vi "DI Coil UI.vi"(8 "error in (no error)":errorcluster, 11 "Node Ptr":T2 format="%.0x") -> (0 "error out":errorcluster)   [LabVIEW 2020, in "Modbus Master System Explorer.lvlib"]
uses:
  Modbus Master System Explorer.lvlib
  <vilib>/NI VeriStand/Custom Device API/Custom Device Item Ref.ctl
  SubVIs/Radix.ctl
  <vilib>/NI VeriStand/Custom Device API/Custom Device API.lvlib
panel:
  in  "Radix":T1
  in  "Valid?":string
  in  "Address":u16
  in  "Header":cluster{"Section Name":string}={"Section Name"="Discrete Input Settings"}
  in  "Description":string
  in  "Name":string
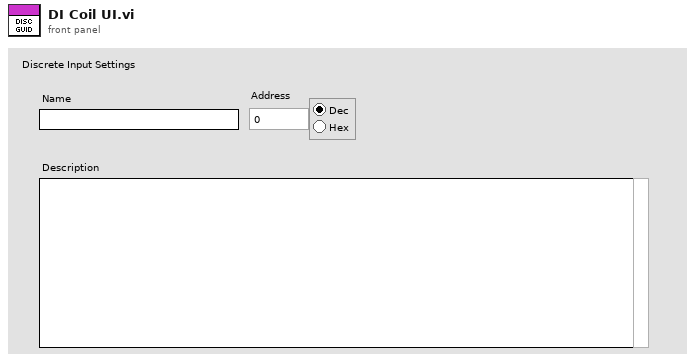
[diagram p1: front panel]
types:
  T1 = typedef "Modbus Master System Explorer.lvlib/Radix.ctl" = enum32{"Decimal", "Hexidecimal"}
  T2 = typedef "Custom Device API.lvlib/Custom Device Item Ref.ctl" = u64
  T3 = typedef "Custom Device API.lvlib/Custom Device Commands.ctl" = enum16{"Default", "Item renamed", "Shutdown", "Dynamic button pressed"}
  T4 = typedef "Custom Device API.lvlib/Custom Device Item Info.ctl" = cluster{"Name":string, "Is Channel":bool, "GUID":string, "Is Waveform":bool}
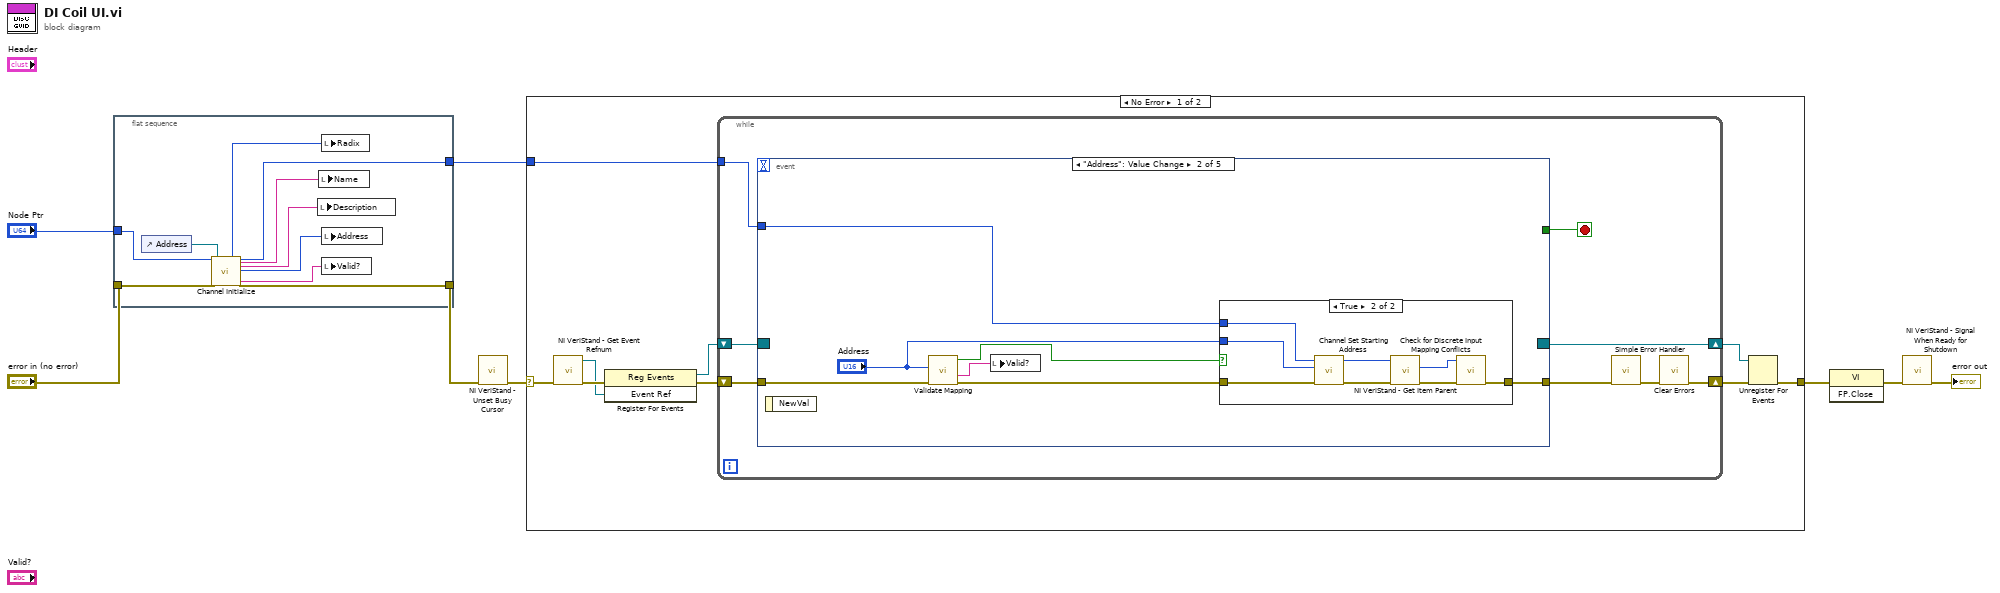
[diagram p0: block diagram]
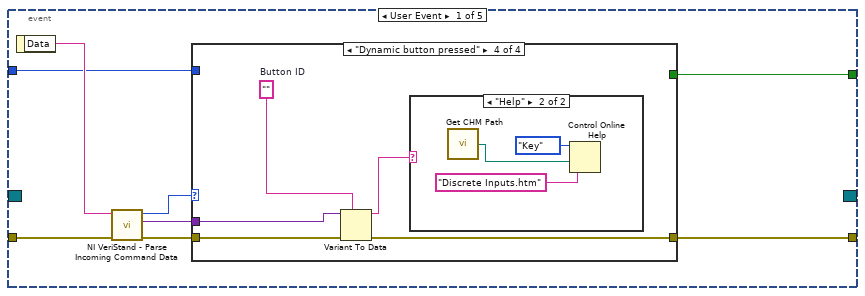
[diagram p2: hidden frame]
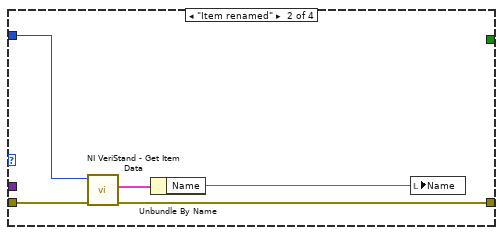
[diagram p4: hidden frame]
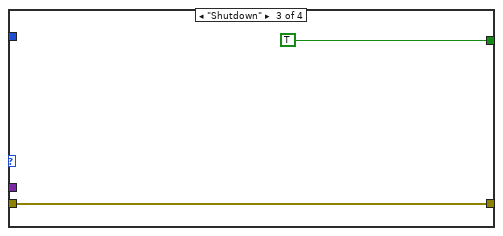
[diagram p5: hidden frame]
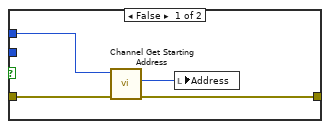
[diagram p7: hidden frame]
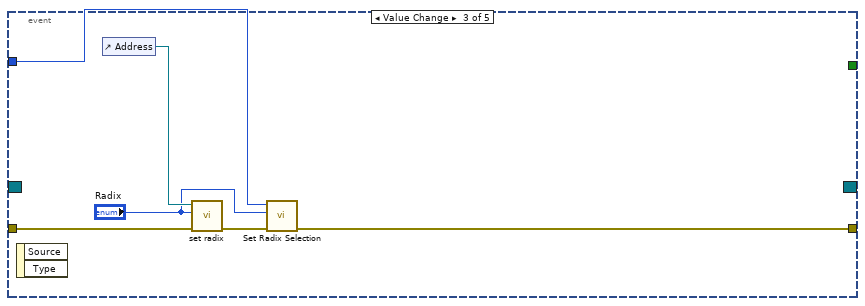
[diagram p8: hidden frame]
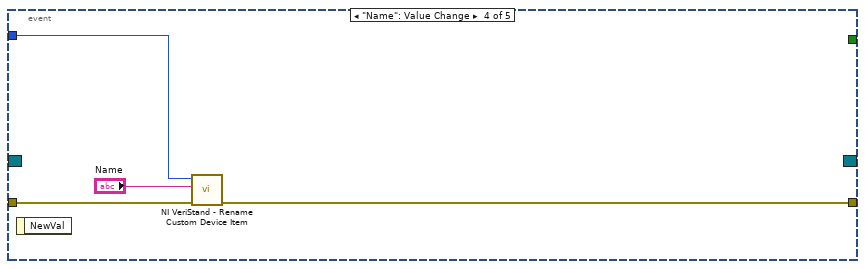
[diagram p9: hidden frame]
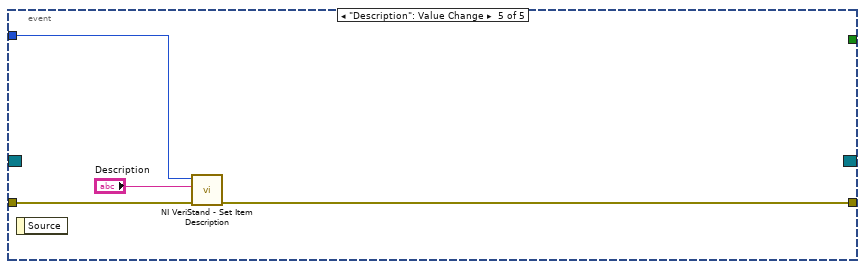
[diagram p10: hidden frame]
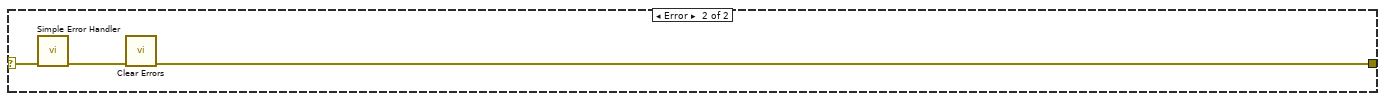
[diagram p11: hidden frame]
diagram:
  n1 = flat-sequence {
    tunnel: "Node Ptr" -> [w12]
    tunnel: [w11] -> w3
    tunnel: "error in (no error)" -> [w10]
    tunnel: [w9] -> w1
    frame #0 {
      n2 = control-ref of="Address"() -> (w17:refnum<vi>)
      n3 = call "Channel Initialize.vi"("Item Ref in"=w12, "error in (no error)"=w10, "Starting Address Ref in"=w17) -> ("Radix"=w18:T1, "Channel Ref out"=w11:T2, "Name"=w15:string, "Description"=w13:string, "Starting Address"=w14:u16, "Status Message"=w16:string, "error out"=w9:errorcluster)  [unwired: 12 in, 6 out]
      n4 = local write "Description"(w13) -> ()
      n5 = local write "Name"(w15) -> ()
      n6 = local write "Radix"(w18) -> ()
      n7 = local write "Address"(w14) -> ()
      n8 = local write "Valid?"(w16) -> ()
    }
  }
  n9 = call <vilib>:"NI VeriStand - Unset Busy Cursor.vi"("error in (no error)"=w1) -> ("error out"=w5:errorcluster)  [unwired: 10 out]
  n10 = case shown="No Error" w5 {
    selector: w5 -> [w19 w95]
    tunnel: [w24 w93] -> w8
    tunnel: w3 -> [w20 _]
    frame No Error {
      n11 = call <vilib>:"NI VeriStand - Get Event Refnum.vi"("error in (no error)"=w19) -> ("error out"=w27:errorcluster, "Event Ref"=w23:refnum<user-event>)  [unwired: 9 out]
      n12 = register-events(error in=w27, w23) -> (reference out=w21:refnum<event-registration>, error out=w22:errorcluster)  [unwired: 1 in]
      n13 = while {
        tunnel: w20 -> [w31]
        shift-right: [w28] -> w25
        shift-left: w22 -> [w34]
        shift-right: [w35] -> w26
        shift-left: w21 -> [w33]
        stop <- w32 stop-if-true
        n14 = event shown="[1] \"Address\": Value Change" {
          selector: w33 -> [_ _ _ _ _]
          dyn-events: [_ _ _ _ _] -> w35
          timeout: _ -> [_ _ _ _ _]
          tunnel: w34 -> [w43 w62 w83 w88 w91]
          tunnel: [w39 _ _ _ _] -> w32
          tunnel: [w38 w64 w80 w87 w90] -> w30
          tunnel: w31 -> [w37 w66 w81 w86 w92]
          event User Event {
            n15 = event-data() -> ("Data"=w42:string)  [unwired: 1 out]
            n16 = call <vilib>:"NI VeriStand - Parse Incoming Command Data.vi"("error in (no error)"=w43, "Incoming data"=w42) -> ("error out"=w41:errorcluster, "Outgoing data"=w36:variant, "Action"=w40:T3)  [unwired: 7 out]
            n17 = case shown="\"Dynamic button pressed\"" w40 {
              tunnel: w41 -> [w44 w49 w50 w56]
              tunnel: [_ _ TRUE _] -> w39
              tunnel: [w44 w46 w50 w53] -> w38
              tunnel: w37 -> [_ w48 _ _]
              tunnel: w36 -> [_ _ _ w55]
              frame "Default", Default {
              }
              frame "Item renamed" {
                n18 = call <vilib>:"NI VeriStand - Get Item Data.vi"("error in (no error)"=w49, "Item Ref in"=w48) -> ("error out"=w46:errorcluster, "Item Info"=w47:T4)  [unwired: 8 out]
                n19 = Unbundle By Name(w47) -> ("Name"=w45:string)
                n20 = local write "Name"(w45) -> ()
              }
              frame "Shutdown" {
              }
              frame "Dynamic button pressed" {
                w54 = ""  # Button ID
                n21 = Variant To Data(error in=w56, type=w54, Variant=w55) -> (data=w52:string, error out=w53:errorcluster)
                n22 = case shown="\"Help\"" w52 {
                  frame Default {
                  }
                  frame "Help" {
                    n23 = call "Get CHM Path.vi"() -> ("appended path"=w59:path)
                    n24 = Control Online Help(2:w59, 3:"Discrete Inputs.htm" ("String to search for"), 4:enum16{"Contents", "Key", "Close"}."Key" ("Operation")) -> ()  [unwired: 1 in, 1 out]
                  }
                }
              }
            }
          }
          event "Address": Value Change {
            n25 = event-data() -> ()  [unwired: 2 out]
            n26 = call "Validate Mapping.vi"("error in (no error)"=w62, "Mapping"="Address") -> ("error out"=w61:errorcluster, "Status Message"=w60:string, "Valid?"=w63:bool)  [unwired: 7 in]
            n27 = local write "Valid?"(w60) -> ()
            n28 = case shown="True" w63 {
              tunnel: w66 -> [w68 w78]
              tunnel: "Address" -> [_ w77]
              tunnel: w61 -> [w70 w76]
              tunnel: [w69 w72] -> w64
              frame False {
                n29 = call "Channel Get Starting Address.vi"("error in (no error)"=w70, "Item Ref in"=w68) -> ("error out"=w69:errorcluster, "Value"=w67:u16)  [unwired: 7 in, 1 out]
                n30 = local write "Address"(w67) -> ()
              }
              frame True {
                n31 = call "Channel Set Starting Address.vi"("error in (no error)"=w76, "Value"=w77, "Item Ref in"=w78) -> ("error out"=w75:errorcluster, "Item Ref out"=w71:T2)  [unwired: 7 in]
                n32 = call <vilib>:"NI VeriStand - Get Item Parent.vi"("error in (no error)"=w75, "Item Ref in"=w71) -> ("error out"=w73:errorcluster, "Parent Ref"=w74:T2)  [unwired: 6 in, 2 out]
                n33 = call "Check for Discrete Input Mapping Conflicts.vi"("error in (no error)"=w73, "Coiil Group Ref in"=w74) -> ("error out"=w72:errorcluster)  [unwired: 6 in, 3 out]
              }
            }
          }
          event Value Change {
            n34 = event-data() -> ()  [unwired: 3 out]
            n35 = control-ref of="Address"() -> (w84:refnum<vi>)
            n36 = call "set radix.vi"("error in (no error)"=w83, "Radix"="Radix", "Digital in"=w84) -> ("error out"=w82:errorcluster)  [unwired: 8 in]
            n37 = call "Set Radix Selection.vi"("error in (no error)"=w82, "Radix"="Radix", "Item Ref in"=w81) -> ("error out"=w80:errorcluster)  [unwired: 7 in, 1 out]
          }
          event "Name": Value Change {
            n38 = event-data() -> ()  [unwired: 2 out]
            n39 = call <vilib>:"NI VeriStand - Rename Custom Device Item.vi"("error in (no error)"=w88, "New Name"="Name", "Item Ref in"=w86) -> ("error out"=w87:errorcluster)  [unwired: 1 in, 7 out]
          }
          event "Description": Value Change {
            n40 = event-data() -> ()  [unwired: 2 out]
            n41 = call <vilib>:"NI VeriStand - Set Item Description.vi"("error in (no error)"=w91, "Description"="Description", "Item Ref in"=w92) -> ("error out"=w90:errorcluster)  [unwired: 8 out]
          }
        }
        n42 = call <vilib>:"Simple Error Handler.vi"("error in (no error)"=w30) -> ("error out"=w29:errorcluster)  [unwired: 1 in, 7 out]
        n43 = call <vilib>:"Clear Errors.vi"("error in (no error)"=w29) -> ("error out"=w28:errorcluster)  [unwired: 1 in, 5 out]
      }
      n44 = Unregister For Events(event registration refnum=w26, error in=w25) -> (error out=w24:errorcluster)
    }
    frame Error {
      n45 = call <vilib>:"Simple Error Handler.vi"("error in (no error)"=w95) -> ("error out"=w94:errorcluster)  [unwired: 1 in, 7 out]
      n46 = call <vilib>:"Clear Errors.vi"("error in (no error)"=w94) -> ("error out"=w93:errorcluster)  [unwired: 1 in, 5 out]
    }
  }
  n47 = invoke class="VI" method="FP.Close"(error in=w8) -> (error out=w7:errorcluster)  [unwired: 2 in, 2 out]
  n48 = call <vilib>:"NI VeriStand - Signal When Ready for Shutdown.vi"("error in (no error)"=w7) -> ("error out"=→"error out":errorcluster)  [unwired: 10 out]
